vi "Setup.vi"(7 "Emit Status Messages (F)":bool, 8 "error in (no error)":errorcluster, 11 "Pub Sub Message Channel in":refnum<class "Pub Sub Message Channel.lvclass">) -> (0 "error out":errorcluster, 3 "Pub Sub Message Channel out":refnum<class "Pub Sub Message Channel.lvclass">)   [LabVIEW 2020, in "Actor Pub Sub Channels.lvlib" / "Pub Sub Message Channel.lvclass"]
uses:
  Pub Sub Message Channel.lvclass
  Pub Sub Message Channel.lvclass/Pub Sub Message Channel.ctl
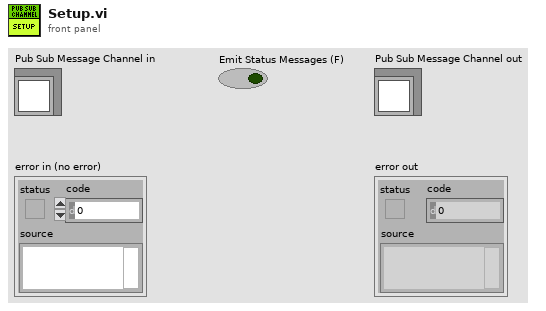
[diagram p1: front panel]
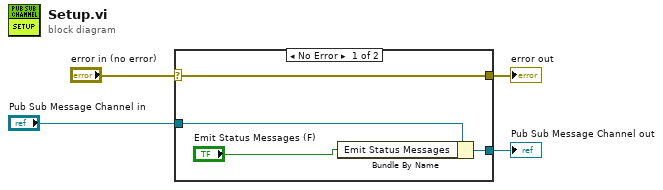
[diagram p0: block diagram]
diagram:
  n1 = case shown="No Error" "error in (no error)" {
    selector: "error in (no error)" -> [w7 w10]
    tunnel: [w7 w10] -> w3
    tunnel: [w6 w9] -> w1
    tunnel: "Pub Sub Message Channel in" -> [w8 w9]
    frame No Error {
      n2 = Bundle By Name(cluster=w8, "Emit Status Messages"="Emit Status Messages (F)") -> (w6:refnum<class "Pub Sub Message Channel.lvclass">)
    }
    frame Error {
    }
  }
  "error out" <- w3
  "Pub Sub Message Channel out" <- w1
